vi "公式节点.vi"() -> ()   [LabVIEW 2017]
panel:
  out "取整后":dbl
  out "取整前":dbl
  in  "停止":bool
  in  "身高":dbl
  in  "体重":dbl
  out "字符串":string
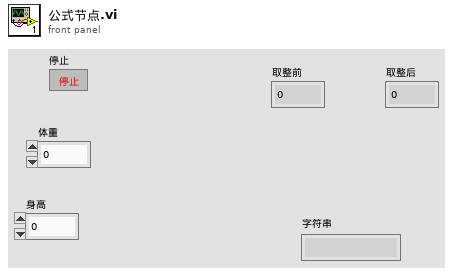
[diagram p1: front panel]
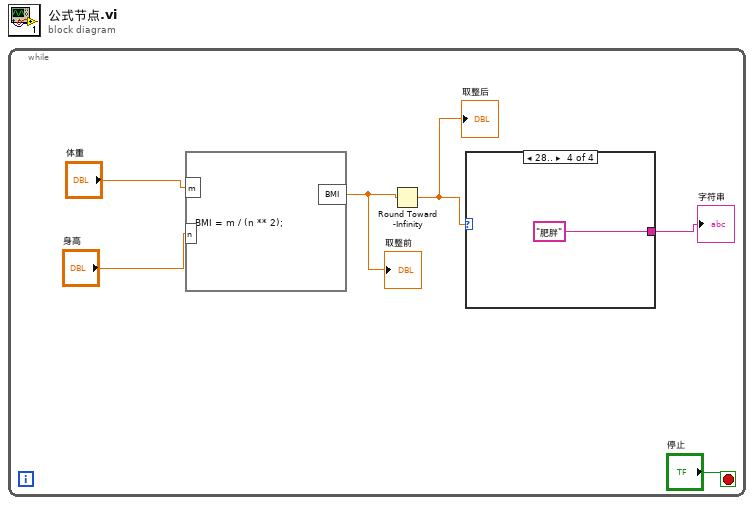
[diagram p0: block diagram]
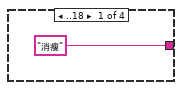
[diagram p2: hidden frame]
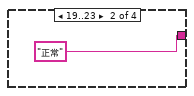
[diagram p3: hidden frame]
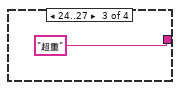
[diagram p4: hidden frame]
diagram:
  n1 = while {
    stop <- "停止" stop-if-true
    n2 = formula code="BMI = m / (n ** 2);"("m"="体重", "n"="身高") -> ("BMI"=w3:dbl)
    "取整前" <- w3
    n3 = Round Toward -Infinity(1:w3) -> (0:w4:dbl)
    "取整后" <- w4
    n4 = case shown="28.." w4 {
      tunnel: ["消瘦" "正常" "超重" "肥胖"] -> w5
      frame ..18 {
      }
      frame 19..23 {
      }
      frame 24..27 {
      }
      frame 28.. {
      }
    }
    "字符串" <- w5
  }
